vi "AUTO_V_MANUAL_CONFIGURATION.vi"(4 "error in":errorcluster, 5 "input path":path=path "C:/Git/Rad-Effects-Test-Software/Python Scripts", 6 "Run Data SubPanel Input":T6, 7 "config file inputs":T5 {"Oscilloscope Configuration Input Array"."vertical coupling" items=["AC", "DC", "Ground"]}) -> (0 "error out":errorcluster, 1 "JSON CONFIGURED?":bool=TRUE, 2 "Run Data Output":T7, 3 "Instrument Configuration Clusters":T4 {"Oscilloscope Configuration Input Array"."vertical coupling" items=["AC", "DC", "Ground"]})   [LabVIEW 2019]
uses:
  Controls/DataBlockControl.ctl
  Controls/VISA_power_Control.ctl
  Controls/RFBlockControl.ctl
  <instrlib>/niScope/Controls/niScope vertical coupling.ctl
panel:
  in  "Run Data Information":T6
  in  "Manual Mode":bool
  in  "Select Configuration":bool
  in  "Config File Selection":u16(ring)=4 items=["ADMV1013s_config", "ADMV1355_config", "ADMV1455_config", "ADMV8818_config", "ADRF6780_config", "EXPERIMENTAL2_config", "EXPERIMENTAL_config"]
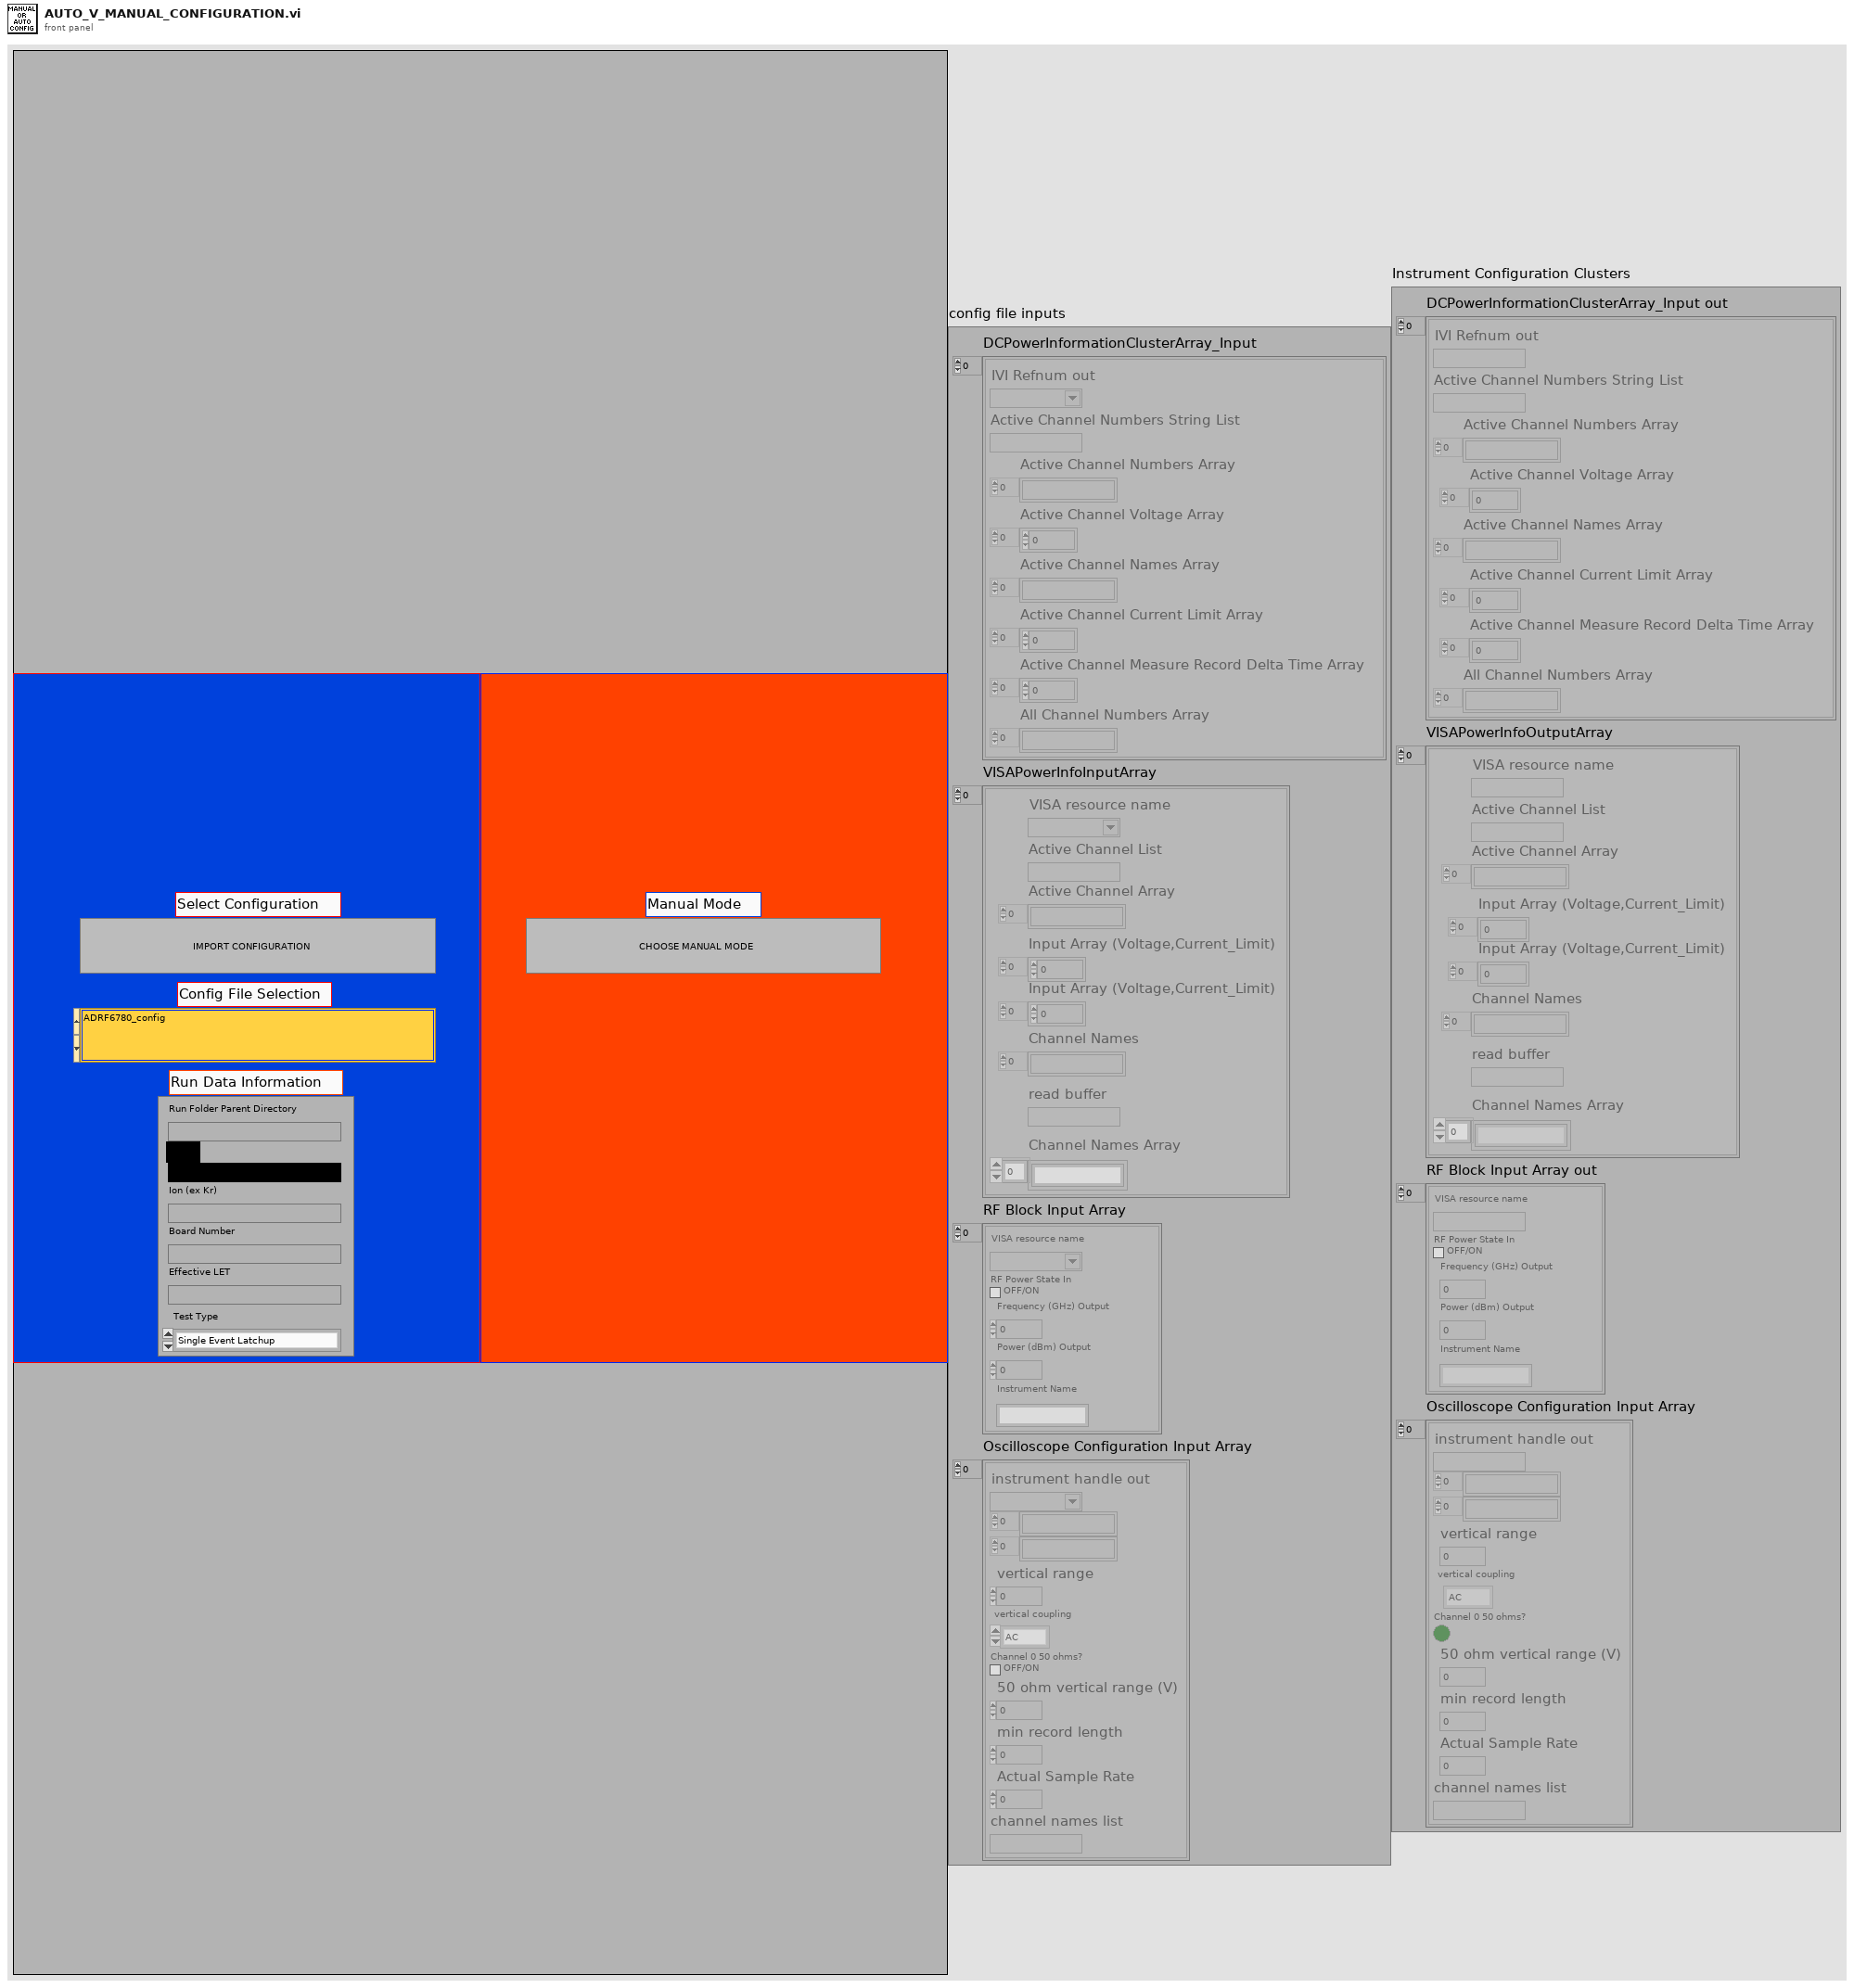
[diagram p1: front panel]
types:
  T1 = typedef "VISA_power_Control.ctl" = cluster{"VISA resource name":refnum<visa-resource-name>, "Active Channel List":string, "Active Channel Array":string[], "Input Array (Voltage,Current_Limit)":dbl[], "Input Array (Voltage,Current_Limit)":dbl[], "Channel Names":string[], "read buffer":string, "Channel Names Array":string[]}
  T2 = typedef "RFBlockControl.ctl" = cluster{"VISA resource name":refnum<visa-resource-name>, "RF Power State In":bool, "Frequency (GHz) Output":dbl, "Power (dBm) Output":dbl, "Instrument Name":string}
  T3 = typedef "niScope vertical coupling.ctl" = i32
  T4 = cluster{"DCPowerInformationClusterArray_Input out":cluster{"IVI Refnum out":refnum<k15>, "Active Channel Numbers String List":string, "Active Channel Numbers Array":string[], "Active Channel Voltage Array":dbl[], "Active Channel Names Array":string[], "Active Channel Current Limit Array":dbl[], "Active Channel Measure Record Delta Time Array":dbl[], "All Channel Numbers Array":string[]}[], "VISAPowerInfoOutputArray":T1[], "RF Block Input Array out":T2[], "Oscilloscope Configuration Input Array":cluster{"instrument handle out":refnum<k15>, string[], string[], "vertical range":dbl, "vertical coupling":T3, "Channel 0 50 ohms?":bool, "50 ohm vertical range (V)":dbl, "min record length":i32, "Actual Sample Rate":dbl, "channel names list":string}[]}
  T5 = cluster{"DCPowerInformationClusterArray_Input":cluster{"IVI Refnum out":refnum<k15>, "Active Channel Numbers String List":string, "Active Channel Numbers Array":string[], "Active Channel Voltage Array":dbl[], "Active Channel Names Array":string[], "Active Channel Current Limit Array":dbl[], "Active Channel Measure Record Delta Time Array":dbl[], "All Channel Numbers Array":string[]}[], "VISAPowerInfoInputArray":T1[], "RF Block Input Array":T2[], "Oscilloscope Configuration Input Array":cluster{"instrument handle out":refnum<k15>, string[], string[], "vertical range":dbl, "vertical coupling":T3, "Channel 0 50 ohms?":bool, "50 ohm vertical range (V)":dbl, "min record length":i32, "Actual Sample Rate":dbl, "channel names list":string}[]}
  T6 = typedef "DataBlockControl.ctl" = cluster{"Run Folder Parent Directory":path, "DUT":string, "Ion (ex Kr)":string, "Board Number":string, "Effective LET":string, "Test Type":enum16{"Single Event Latchup", "Single Event Transient", "Single Event Upset"}}
  T7 = cluster{"path out":path, string, "Ion (ex Kr)":string, "Board Number":string, "Effective LET":string, "Test Type":enum16{"Single Event Latchup", "Single Event Transient", "Single Event Upset"}}
  T8 = typedef "LVStringsAndValuesArrayTypeDef_U16.ctl" = cluster{"String":string, "Value":u16}[]
  T9 = enum16{"Single Event Latchup", "Single Event Transient", "Single Event Upset"}
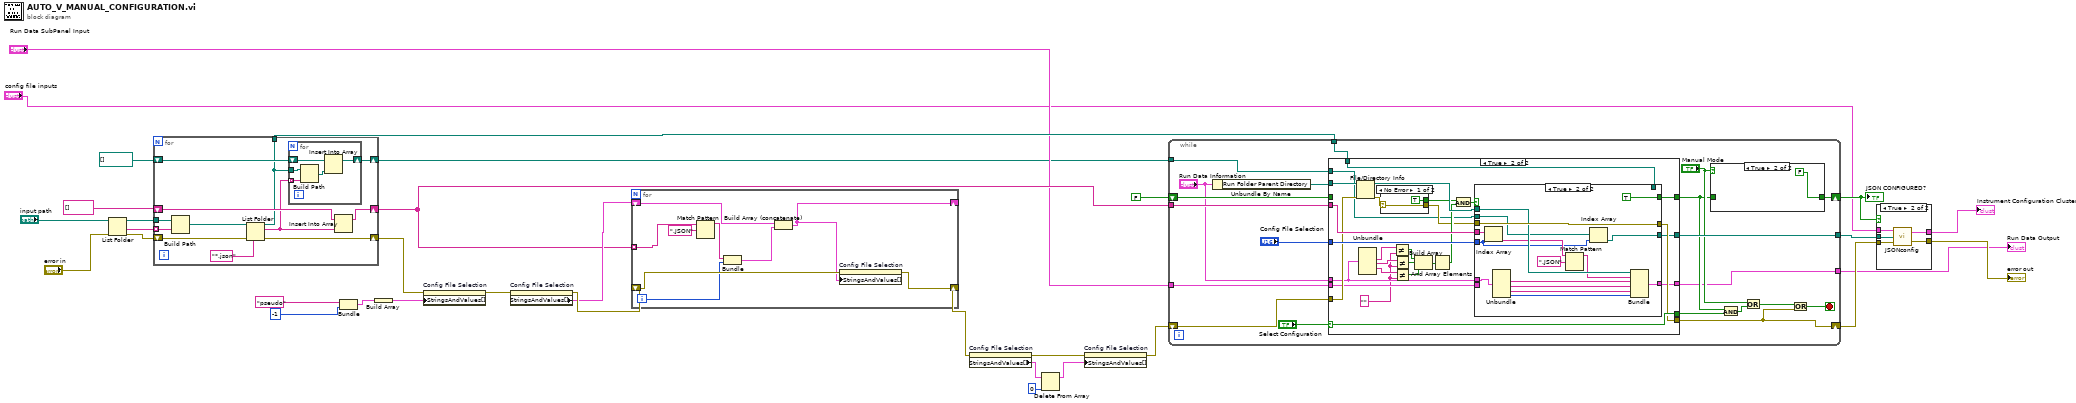
[diagram p0: block diagram]
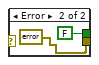
[diagram p5: hidden frame]
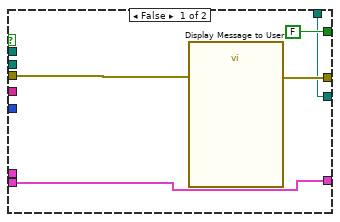
[diagram p6: hidden frame]
diagram:
  n1 = List Folder(path="input path", error in="error in") -> (path out=w21:path, folder names=w22:string[], error out=w20:errorcluster)  [unwired: 2 in, 1 out]
  n2 = for {
    tunnel: w22 -> [w45] mode=indexing
    tunnel: w21 -> [w44]
    shift-right: [w40] -> w16
    shift-left: w20 -> [w42]
    shift-right: [w38] -> w14
    shift-left: string[] [] ("array") -> [w39]
    tunnel: [w34] -> w18
    shift-right: [w36] -> w3
    shift-left: path[] [] -> [w35]
    n3 = Build Path(base path=w44, name or relative path=w45) -> (appended path=w43:path)
    n4 = List Folder(path=w43, pattern="*.json", error in=w42) -> (path out=w34:path, filenames=w37:string[], error out=w40:errorcluster)  [unwired: 1 in, 1 out]
    n5 = for {
      tunnel: w37 -> [w50] mode=indexing
      shift-right: [w47] -> w36
      shift-left: w35 -> [w48]
      tunnel: w34 -> [w46]
      n6 = Build Path(base path=w46, name or relative path=w50) -> (appended path=w49:path)
      n7 = Insert Into Array(array=w48, new element=w49) -> (w47:path[])  [unwired: 1 in]
    }
    n8 = Insert Into Array(array=w39, new element=w37) -> (w38:string[])  [unwired: 1 in]
  }
  n9 = Bundle("concatenated string"="pseudo", -1) -> (w33:cluster{"concatenated string":string, i32})  [unwired: 1 in]
  n10 = Build Array(w33) -> (w30:cluster{"concatenated string":string, i32}[])
  n11 = property on="Config File Selection" class="Ring (strict)"(error in=w16, "StringsAndValues[]"=w30) -> (error out=w29:errorcluster)  [unwired: 1 in, 1 out]
  n12 = property on="Config File Selection" class="Ring (strict)"(error in=w29) -> (error out=w28:errorcluster, "StringsAndValues[]"=w27:T8)  [unwired: 1 in, 1 out]
  n13 = for {
    shift-right: [w58] -> w13
    shift-left: w28 -> [w59]
    shift-right: [w51] -> _
    shift-left: w27 -> [w52]
    tunnel: w14 -> [w55] mode=indexing
    i -> [w56]
    n14 = Match Pattern(string=w55, regular expression=".JSON") -> (before substring=w53:string)  [unwired: 1 in, 3 out]
    n15 = Bundle(w53, w56) -> (w57:cluster{string, i32})  [unwired: 1 in]
    n16 = Build Array (concatenate)(w52, w57) -> (w51:cluster{"String":string, "Value":i32}[])
    n17 = property on="Config File Selection" class="Ring (strict)"(error in=w59, "StringsAndValues[]"=w51) -> (error out=w58:errorcluster)  [unwired: 1 in, 1 out]
  }
  n18 = property on="Config File Selection" class="Ring (strict)"(error in=w13) -> (error out=w10:errorcluster, "StringsAndValues[]"=w12:T8)  [unwired: 1 in, 1 out]
  n19 = Delete From Array(array=w12, index=0) -> (array with subset deleted=w9:T8)  [unwired: 1 in, 1 out]
  n20 = property on="Config File Selection" class="Ring (strict)"(error in=w10, "StringsAndValues[]"=w9) -> (error out=w8:errorcluster)  [unwired: 1 in, 1 out]
  n21 = while {
    shift-right: [w76] -> w26
    shift-left: w8 -> [w78]
    tunnel: w14 -> [w75]
    tunnel: w18 -> [w73]
    tunnel: [w72] -> w25
    shift-right: [w71] -> w5
    shift-left: FALSE -> [w70]
    tunnel: "Run Data SubPanel Input" -> [w64]
    tunnel: [w61] -> w6
    tunnel: w3 -> [w60]
    stop <- w79 stop-if-true
    n22 = Unbundle By Name("Run Data Information") -> ("Run Folder Parent Directory"=w63:path)
    n23 = case shown="True" "Select Configuration" {
      selector: "Select Configuration" -> [w85 w111]
      tunnel: w78 -> [w86 w109]
      tunnel: [w86 w107] -> w76
      tunnel: w75 -> [_ w113]
      tunnel: "Config File Selection" -> [_ w112]
      tunnel: w73 -> [w84 w87]
      tunnel: [w84 w88] -> w72
      tunnel: [w85 w111] -> w66
      tunnel: [w83 w110] -> w67
      tunnel: w70 -> [w83 _]
      tunnel: w63 -> [_ w108]
      tunnel: w64 -> [w82 w106]
      tunnel: "Run Data Information" -> [_ w103]
      tunnel: [w82 w104] -> w61
      tunnel: w60 -> [_ w89]
      frame False {
      }
      frame True {
        w99 = "" ("y")
        n24 = File/Directory Info(path=w108, error in=w109) -> (path out=w105:path, error out=w91:errorcluster)  [unwired: 5 out]
        n25 = Unbundle(w103) -> ("Ion (ex Kr)"=w102:string, "Board Number"=w101:string, "Effective LET"=w100:string)  [unwired: 3 out]
        n26 = case shown="No Error" w91 {
          selector: w91 -> [w114 _]
          tunnel: [TRUE FALSE] -> w92
          tunnel: [w114 errorcluster {"status"=FALSE, "code"=0, "source"=""} ("error IO")] -> w90
          frame No Error {
          }
          frame Error {
          }
        }
        n27 = Not Equal?(x=w102, y=w99) -> (x != y?=w96:bool)
        n28 = Not Equal?(x=w101, y=w99) -> (x != y?=w97:bool)
        n29 = Not Equal?(x=w100, y=w99) -> (x != y?=w98:bool)
        n30 = Build Array(w96, w97, w98) -> (w95:bool[])
        n31 = And Array Elements(Boolean array=w95) -> (logical AND=w94:bool)
        n32 = And(x=w92, y=w94) -> (x .and. y?=w93:bool)
        n33 = case shown="True" w93 {
          tunnel: w113 -> [_ w138]
          tunnel: w112 -> [_ w125]
          tunnel: w89 -> [_ w124]
          tunnel: [FALSE TRUE] -> w110
          tunnel: w90 -> [w121 w136]
          tunnel: [w120 w136] -> w107
          tunnel: w106 -> [w119 _]
          tunnel: w105 -> [_ w135]
          tunnel: w103 -> [_ w134]
          tunnel: [w119 w126] -> w104
          tunnel: [w118 w123] -> w88
          tunnel: w87 -> [w118 _]
          frame False {
            n34 = call "Display Message to User"("error in (no error)"=w121) -> ("error out"=w120:errorcluster)  [unwired: 9 in, 1 out]
          }
          frame True {
            n35 = Index Array(array=w138, index=w125) -> (element=w132:string)
            n36 = Unbundle(w134) -> ("Ion (ex Kr)"=w130:string, "Board Number"=w129:string, "Effective LET"=w128:string, "Test Type"=w127:T9)  [unwired: 2 out]
            n37 = Match Pattern(string=w132, regular expression=".JSON") -> (before substring=w131:string)  [unwired: 1 in, 3 out]
            n38 = Index Array(array=w124, index=w125) -> (element=w123:path)
            n39 = Bundle("path out"=w135, w131, "Ion (ex Kr)"=w130, "Board Number"=w129, "Effective LET"=w128, "Test Type"=w127) -> (w126:T7)  [unwired: 1 in]
          }
        }
      }
    }
    n40 = case shown="True" "Manual Mode" {
      tunnel: [w80 FALSE] -> w71
      tunnel: w67 -> [w80 _]
      frame False {
      }
      frame True {
      }
    }
    n41 = And(x=w67, y=w66) -> (x .and. y?=w69:bool)
    n42 = Or(x="Manual Mode", y=w69) -> (x .or. y?=w65:bool)
    n43 = Or(x=w65, y=w76) -> (x .or. y?=w79:bool)
  }
  "JSON CONFIGURED?" <- w5
  "Run Data Output" <- w6
  n44 = case shown="True" w5 {
    tunnel: "config file inputs" -> [w139 w145]
    tunnel: w26 -> [w140 w144]
    tunnel: w25 -> [_ w143]
    tunnel: [w140 w142] -> w24
    tunnel: [w139 w141] -> w1
    frame False {
    }
    frame True {
      n45 = call "JSONconfig.vi"("error in (no error)"=w144, "file path (use dialog)"=w143, "config file inputs"=w145) -> ("error out"=w142:errorcluster, "Instrument Configuration Clusters"=w141:T4)
    }
  }
  "error out" <- w24
  "Instrument Configuration Clusters" <- w1
